vi "Get QueueByNumber.vi"(10 "Priority Level":i32, 11 "PriorityMessageQueue in":refnum<class "PriorityMessageQueue.lvclass">) -> (2 "Message Queue":refnum<queue>, 3 "PriorityMessageQueue out":refnum<class "PriorityMessageQueue.lvclass">)   [LabVIEW 2009, in "LapDog.Messaging.v2.lvlib" / "PriorityMessageQueue.lvclass"]
uses:
  PriorityMessageQueue.lvclass
  MessageObject/Message.lvclass
  PriorityMessageQueue.lvclass/PriorityMessageQueue.ctl
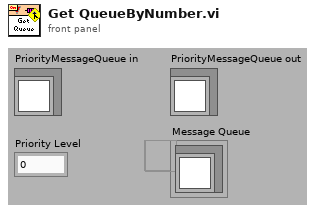
[diagram p1: front panel]
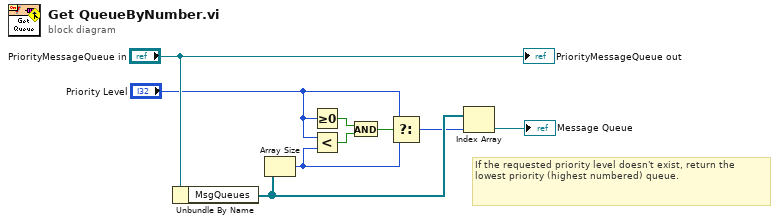
[diagram p0: block diagram]
diagram:
  # "If the requested priority level doesn't exist, return the lowest priority (highest numbered) queue."
  n1 = Unbundle By Name("PriorityMessageQueue in") -> ("MsgQueues"=w7:refnum<queue>[])
  n2 = Array Size(array=w7) -> (size(s)=w5:i32)
  n3 = Greater Or Equal To 0?(x="Priority Level") -> (x >= 0?=w4:bool)
  n4 = Less?(x="Priority Level", y=w5) -> (x < y?=w3:bool)
  n5 = And(x=w4, y=w3) -> (x .and. y?=w2:bool)
  n6 = Select(t="Priority Level", s=w2, f=w5) -> (s? t:f=w1:i32)
  n7 = Index Array(array=w7, index=w1) -> (element=→"Message Queue":refnum<queue>)
  "PriorityMessageQueue out" <- "PriorityMessageQueue in"
